vi "Set Value.vi"(8 "error in (no error)":errorcluster, 10 "Variant":variant, 11 "Refnum Value Source in":refnum<class "Path Ctrl Refnum.lvclass">) -> (0 "error out":errorcluster, 3 "Refnum Value Source out":refnum<class "Path Ctrl Refnum.lvclass">)   [LabVIEW 2020, in "Composed Columns.lvlib" / "Path Ctrl Refnum.lvclass"]
uses:
  Path Ctrl Refnum.lvclass
  Ctrl Renum Value Source Class/Ctrl Refnum Value Source.lvclass
  <vilib>/Utility/Data Type/NI_Data Type.lvlib
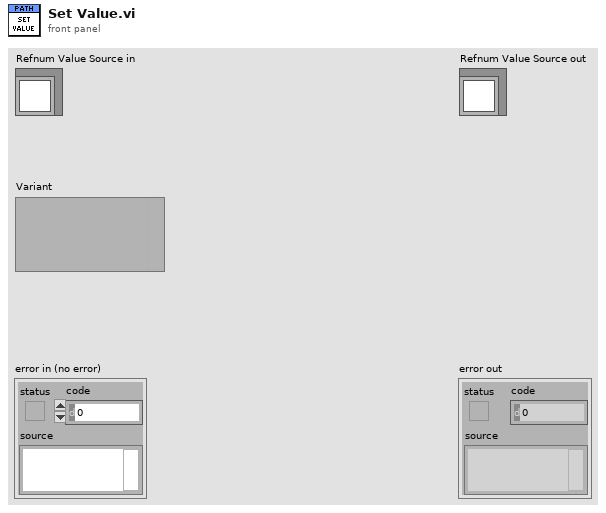
[diagram p1: front panel]
types:
  T1 = typedef "NI_Data Type.lvlib/Data Type.ctl" = enum8{"Invalid Type", "Void", "I8", "I16", "I32", "I64", "U8", "U16", "U32", "U64", "Single Float", "Double Float", "Extended Float", "Single Complex", "Double Complex", "Extended Complex", "Enum U8", "Enum U16", "Enum U32", "Enum U64", "Single Float With Unit", "Double Float With Unit", "Extended Float With Unit", "Single Complex with Unit", "Double Complex with Unit", "Extended Complex with Unit", "Boolean", "String", "Path", "Picture", "Tag", "Array", "Cluster", "Variant", "LV Variant", "Waveform", "Timestamp", "Digital Waveform", "Digital Data", "ExpressData", "Refnum", "External Data", "VI", "Poly VI", "LabVIEW Class Instance", "Fixed Point", "Set Collection", "Map Collection"}
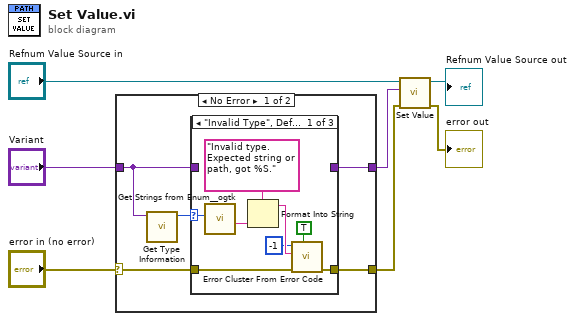
[diagram p0: block diagram]
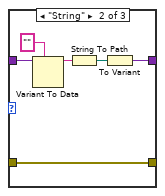
[diagram p2: hidden frame]
diagram:
  n1 = case shown="No Error" "error in (no error)" {
    selector: "error in (no error)" -> [w9 w29]
    tunnel: "Variant" -> [w11 _]
    tunnel: [w10 _] -> w4
    tunnel: [w8 w29] -> w2
    frame No Error {
      n2 = call <vilib>:"Get Type Information.vi"("variant"=w11) -> ("type"=w12:T1)  [unwired: 6 in, 4 out]
      n3 = case shown="\"Invalid Type\", Default" w12 {
        selector: w12 -> [w20 _ _]
        tunnel: w11 -> [_ w26 w28]
        tunnel: [_ w22 w28] -> w10
        tunnel: w9 -> [w13 w21 w27]
        tunnel: [w17 w21 w27] -> w8
        frame "Invalid Type", Default {
          n4 = call <userlib>:"Get Strings from Enum__ogtk.vi"("Enum"=w20) -> ("String Value"=w18:string)  [unwired: 7 in, 3 out]
          n5 = Format Into String(format string="Invalid type. Expected string or path, got %S.", w18) -> (resulting string=w16:string)  [unwired: 2 in, 1 out]
          n6 = call <vilib>:"Error Cluster From Error Code.vi"("show call chain? (False)"=TRUE, "error in (no error)"=w13, "error message (\"\")"=w16, "error code (0)"=-1) -> ("error out"=w17:errorcluster)  [unwired: 5 in]
        }
        frame "String" {
          n7 = Variant To Data(type="", Variant=w26) -> (data=w24:string)  [unwired: 1 in, 1 out]
          n8 = String To Path(string=w24) -> (path=w23:path)
          n9 = To Variant(anything=w23) -> (Variant=w22:variant)
        }
        frame "Path" {
        }
      }
    }
    frame Error {
    }
  }
  n10 = call-parent "Set Value.vi"("error in (no error)"=w2, "Variant"=w4, "Refnum Value Source in"="Refnum Value Source in") -> ("error out"=→"error out":errorcluster, "Refnum Value Source out"=→"Refnum Value Source out":refnum<class "Path Ctrl Refnum.lvclass">)  [unwired: 7 in]
